vi "Configure Numeric Control.vi"(8 "error in":errorcluster, 10 "control":refnum<vi>, 11 "Value in":refnum<class "Value.lvclass">) -> (0 "error out":errorcluster, 3 "Value out":refnum<class "Value.lvclass">)   [LabVIEW 2020, in "Value.lvlib" / "Value.lvclass"]
doc: "Set the format, precision and limits of the control from the value metadata"
uses:
  Value/Value/Value.lvclass
  Value/Value/Value.lvclass/Value.ctl
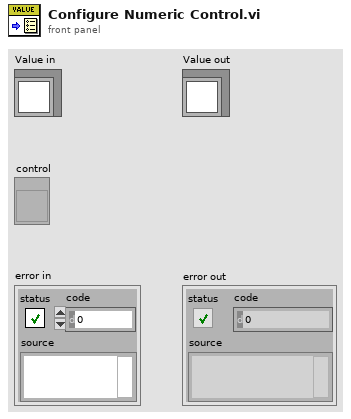
[diagram p1: front panel]
types:
  T1 = typedef "Value.lvlib/Display Metadata.ctl" = cluster{"Limit Low":dbl, "Limit High":dbl, "Description":string, "Units":string, "Precision":i32, "Form":enum32{"Default", "String", "Binary", "Decimal", "Hex", "Exponential", "Engineering"}}
  T2 = enum32{"Default", "String", "Binary", "Decimal", "Hex", "Exponential", "Engineering"}
  T3 = typedef "Value.lvlib/Control Metadata.ctl" = cluster{"Limit Low":dbl, "Limit High":dbl, "Min Step":dbl}
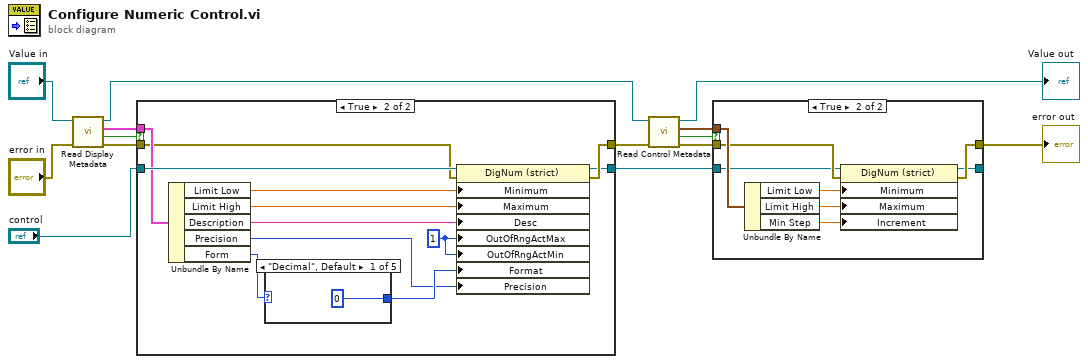
[diagram p0: block diagram]
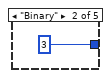
[diagram p4: hidden frame]
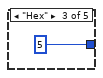
[diagram p5: hidden frame]
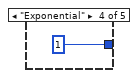
[diagram p6: hidden frame]
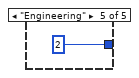
[diagram p7: hidden frame]
diagram:
  n1 = call "Read Display Metadata.vi"("error in"="error in", "Value in"="Value in") -> ("error out"=w10:errorcluster, "has display metadata?"=w7:bool, "display metadata"=w11:T1, "Value out"=w8:refnum<class "Value.lvclass">)  [unwired: 6 in]
  n2 = case shown="True" w7 {
    tunnel: "control" -> [w15 w26]
    tunnel: w11 -> [_ w25]
    tunnel: w10 -> [w16 w24]
    tunnel: [w16 w18] -> w9
    tunnel: [w15 w17] -> w1
    frame False {
    }
    frame True {
      w21 = u8 1 ("Response to Value Outside Limits:Maximum")
      n3 = Unbundle By Name(w25) -> ("Limit Low"=w28:dbl, "Limit High"=w27:dbl, "Description"=w22:string, "Precision"=w19:i32, "Form"=w23:T2)
      n4 = case shown="\"Decimal\", Default" w23 {
        tunnel: [u8 0 u8 3 u8 5 u8 1 u8 2] -> w20
        frame "Decimal", Default {
        }
        frame "Binary" {
        }
        frame "Hex" {
        }
        frame "Exponential" {
        }
        frame "Engineering" {
        }
      }
      n5 = property on="Property Node" class="DigNum (strict)"(reference=w26, error in=w24, "Minimum"=w28, "Maximum"=w27, "Desc"=w22, "OutOfRngActMax"=w21, "OutOfRngActMin"=w21, "Format"=w20, "Precision"=w19) -> (reference out=w17:refnum<vi>, error out=w18:errorcluster)
    }
  }
  n6 = call "Read Control Metadata.vi"("error in"=w9, "Value in"=w8) -> ("error out"=w6:errorcluster, "has control metadata?"=w5:bool, "control metadata"=w4:T3, "Value out"=→"Value out":refnum<class "Value.lvclass">)  [unwired: 6 in]
  n7 = case shown="True" w5 {
    tunnel: w4 -> [_ w41]
    tunnel: w6 -> [w35 w40]
    tunnel: [w35 w39] -> w2
    tunnel: w1 -> [w34 w37]
    tunnel: [w34 w36] -> _
    frame False {
    }
    frame True {
      n8 = Unbundle By Name(w41) -> ("Limit Low"=w43:dbl, "Limit High"=w42:dbl, "Min Step"=w38:dbl)
      n9 = property on="Property Node" class="DigNum (strict)"(reference=w37, error in=w40, "Minimum"=w43, "Maximum"=w42, "Increment"=w38) -> (reference out=w36:refnum<vi>, error out=w39:errorcluster)
    }
  }
  "error out" <- w2
